vi "Controller.vi"() -> ()   [LabVIEW 2018]
uses:
  <vilib>/Platform/TimedLoop/XDataNode/timing_clust.ctl
  <vilib>/Platform/TimedLoop/XDataNode/nitl_modes.ctl
  <vilib>/Platform/TimedLoop/XDataNode/wakeup.ctl
  <vilib>/Modbus/master/Create Master Instance (TCP).vi
  <vilib>/Modbus/slave/Create Slave Instance (TCP).vi
  <vilib>/Modbus/master/Modbus Master.lvclass
  <vilib>/Platform/TimedLoop/XDataNode/XDataNode.xnode
  <vilib>/Platform/TimedLoop/XDataNode/XDNodeRunTimeDep.lvlib
  <vilib>/Modbus/slave/Modbus Slave.lvclass
panel:
  in  "stop":bool
  out "BPCS-10TY100":dbl format="%.2f"
  out "BPCS-10AY300":dbl
  out "BPCS-SIM-TX-ARRAY":dbl[](array[numeric])
  out "BPCS-10Y200":dbl format="%.2f"
  out "HMI-10HIC100":dbl
  out "HMI-10TIC100-SP":dbl
  out "HMI-10TIC100-KPID":dbl[](array[numeric])
  out "HMI-10HIC200":dbl
  out "HMI-10LIC200-SP":dbl
  out "HMI-10LIC200-KPID":dbl[](array[numeric])
  out "HMI-10HIC300":dbl
  out "HMI-10TIC100_MA":bool
  out "HMI-10LIC200_MA":bool
  out "SIS-BPCS-RX-Array":bool[](array[boolean])
  out "SIS-10SDV501":bool
  out "SIS-10SDV500":bool
  out "SIS-10SDV502":bool
  out "BPCS-10LI200":dbl
  out "SIM-BPCS-RX-ARRAY":dbl[](array[numeric])
  out "BPCS-10TI100":dbl
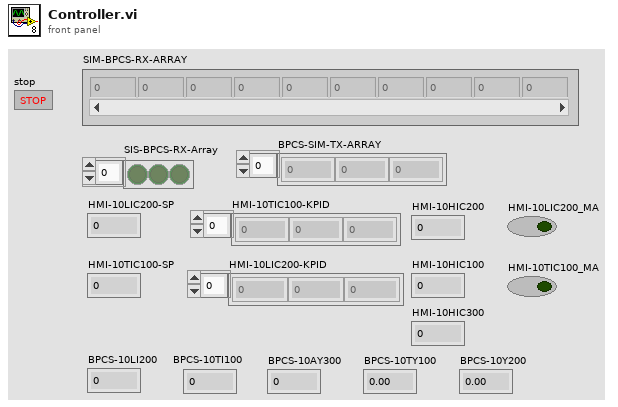
[diagram p1: front panel]
types:
  T1 = typedef "XDNodeRunTimeDep.lvlib/timing_clust.ctl" = cluster{"Expected End [f-1]":u64, "Actual End [f-1]":u64, "Finished Late? [f-1]":bool, "Expected End [i-1]":u64, "Actual End [i-1]":u64, "Finished Late? [i-1]":bool, "Expected Start [i]":u64, "Actual Start [i]":u64, "Expected Start [f]":u64, "Actual Start [f]":u64, "Source Name":string, "Structure Name":string, "Period":i64, "Deadline":i64, "Offset":i64, "Start":i64, "Priority":i32, "Timeout":i32, "Mode":T2, "Wakeup Reason":T3, "Error":errorcluster, "Source Type":string, "Secondary Source Type":string, "Global End Time":u64, "Global Start Time":u64, "Frame Duration":u64, "Iteration Duration":u64, "Assigned CPU":i32, "I/O Scan Engine Mode":u32}
  T2 = typedef "XDNodeRunTimeDep.lvlib/nitl_modes.ctl" = enum32{"No Change", "Process missed periods, maintain original phase", "Discard missed periods, maintain original phase", "Process missed periods, ignore original phase", "Discard missed periods, ignore original phase"}
  T3 = typedef "XDNodeRunTimeDep.lvlib/wakeup.ctl" = enum32{"Normal", "Aborted", "Asynchronous wakeup", "Timing source error", "Timed loop error", "Timeout"}
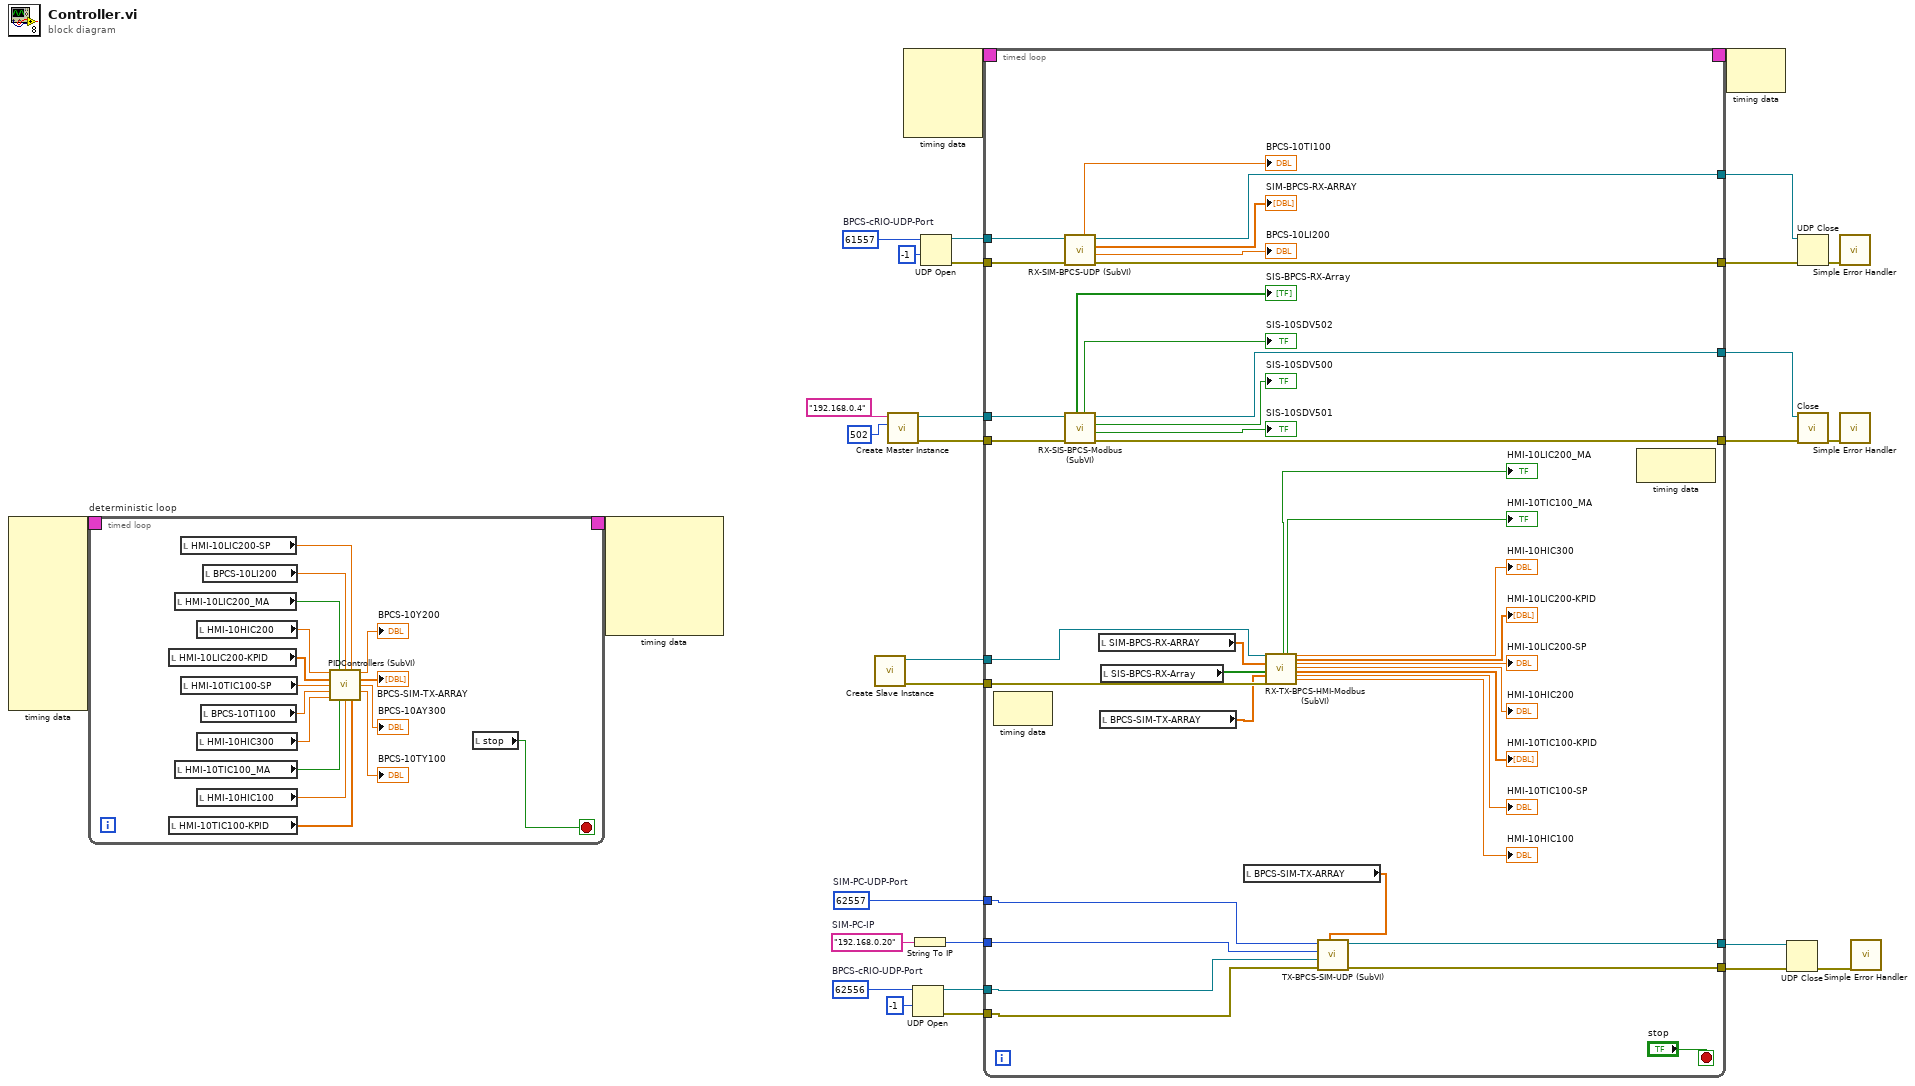
[diagram p0: block diagram]
diagram:
  w11 = u16 62556  # BPCS-cRIO-UDP-Port
  w9 = u16 62557  # SIM-PC-UDP-Port
  w12 = "192.168.0.20"  # SIM-PC-IP
  w28 = u16 61557  # BPCS-cRIO-UDP-Port
  n1 = node-c288 ("Input Node")() -> (w2:T1)  [unwired: 10 in]
  n2 = timed-loop "deterministic loop" {
    timing: w2 -> [_]
    timing-out: [_] -> w1
    stop <- w31 stop-if-true
    n3 = local read "HMI-10LIC200-KPID"() -> (w42:dbl[])
    n4 = local read "HMI-10TIC100-KPID"() -> (w36:dbl[])
    n5 = local read "HMI-10LIC200_MA"() -> (w44:bool)
    n6 = local read "HMI-10TIC100_MA"() -> (w38:bool)
    n7 = local read "HMI-10LIC200-SP"() -> (w46:dbl)
    n8 = local read "HMI-10TIC100-SP"() -> (w41:dbl)
    n9 = local read "HMI-10HIC200"() -> (w43:dbl)
    n10 = local read "HMI-10HIC300"() -> (w39:dbl)
    n11 = local read "HMI-10HIC100"() -> (w37:dbl)
    n12 = local read "BPCS-10TI100"() -> (w40:dbl)
    n13 = local read "BPCS-10LI200"() -> (w45:dbl)
    n14 = call "PIDControllers (SubVI).vi"("HMI-10HIC200"=w43, "HMI-10LIC200_MA"=w44, "BPCS-10LI200"=w45, "HMI-10LIC200-SP"=w46, "HMI-10LIC200-KPID"=w42, "HMI-10TIC100-SP"=w41, "BPCS-10TI100"=w40, "HMI-10HIC300"=w39, "HMI-10TIC100_MA"=w38, "HMI-10HIC100"=w37, "HMI-10TIC100-KPID"=w36) -> ("BPCS-10Y200"=→"BPCS-10Y200":dbl, "BPCS-SIM-TX-ARRAY"=→"BPCS-SIM-TX-ARRAY":dbl[], "BPCS-10AY300"=→"BPCS-10AY300":dbl, "BPCS-10TY100"=→"BPCS-10TY100":dbl)  [unwired: 1 in]
    n15 = local read "stop"() -> (w31:bool)
  }
  n16 = node-c288 ("Output Node")(w1) -> ()  [unwired: 6 out]
  n17 = call-poly <vilib>:"Create Slave Instance.vi"() -> ("error out"=w13:errorcluster, "TCP slave instance"=w14:refnum<class "Modbus Slave.lvclass">)  [unwired: 10 in]
  n18 = call-poly <vilib>:"Create Master Instance.vi"("port (502)"=u16 502, "address"="192.168.0.4") -> ("error out"=w18:errorcluster, "TCP master instance"=w19:refnum<class "Modbus Master.lvclass">)  [unwired: 8 in]
  n19 = node-c288() -> (w30:T1)  [unwired: 4 in]
  n20 = UDP Open(9:-1 ("timeout ms (25000)"), 11:w11) -> (port=w7:refnum<k16>, 0:w6:errorcluster)  [unwired: 3 in, 1 out]
  n21 = String To IP(1:w12) -> (0:w8:u32)
  n22 = UDP Open(9:-1 ("timeout ms (25000)"), 11:w28) -> (port=w26:refnum<k16>, 0:w25:errorcluster)  [unwired: 3 in, 1 out]
  n23 = timed-loop {
    timing: w30 -> [_]
    timing-out: [_] -> w29
    tunnel: w26 -> [w85]
    tunnel: w25 -> [w84]
    tunnel: [w83] -> w23
    tunnel: [w82] -> w22
    tunnel: w19 -> [w78]
    tunnel: w18 -> [w77]
    tunnel: [w76] -> w16
    tunnel: [w75] -> w15
    tunnel: w14 -> [w71]
    tunnel: w13 -> [w70]
    tunnel: w9 -> [w57]
    tunnel: w8 -> [w56]
    tunnel: w7 -> [w55]
    tunnel: w6 -> [w54]
    tunnel: [w53] -> w4
    tunnel: [w52] -> w3
    stop <- "stop" stop-if-true
    n24 = node-c288() -> ()  [unwired: 1 in, 1 out]
    n25 = call "RX-SIM-BPCS-UDP (SubVI).vi"("error in (no error)"=w84, "UDP Network Connection in"=w85) -> ("error out"=w82:errorcluster, "BPCS-10LI200"=→"BPCS-10LI200":dbl, "SIM-BPCS-RX-ARRAY"=→"SIM-BPCS-RX-ARRAY":dbl[], "UDP Network Connection out"=w83:refnum<k16>, "BPCS-10TI100"=→"BPCS-10TI100":dbl)  [unwired: 5 in]
    n26 = call "RX-SIS-BPCS-Modbus (SubVI).vi"("error in (no error)"=w77, "Modbus Master in"=w78) -> ("error out"=w75:errorcluster, "SIS-10SDV501"=→"SIS-10SDV501":bool, "SIS-10SDV500"=→"SIS-10SDV500":bool, "Modbus Master out"=w76:refnum<class "Modbus Master.lvclass">, "SIS-10SDV502"=→"SIS-10SDV502":bool, "SIS-BPCS-RX-Array"=→"SIS-BPCS-RX-Array":bool[])  [unwired: 4 in]
    n27 = local read "SIM-BPCS-RX-ARRAY"() -> (w68:dbl[])
    n28 = local read "BPCS-SIM-TX-ARRAY"() -> (w51:dbl[])
    n29 = local read "SIS-BPCS-RX-Array"() -> (w67:bool[])
    n30 = local read "BPCS-SIM-TX-ARRAY"() -> (w50:dbl[])
    n31 = call "RX-TX-BPCS-HMI-Modbus (SubVI).vi"("Modbus Slave in"=w71, "SIM-BPCS-RX-ARRAY"=w68, "SIS-BPCS-RX-Array"=w67, "BPCS-SIM-TX-ARRAY"=w51, "error in (no error)"=w70) -> ("HMI-10LIC200_MA"=→"HMI-10LIC200_MA":bool, "HMI-10TIC100_MA"=→"HMI-10TIC100_MA":bool, "HMI-10HIC300"=→"HMI-10HIC300":dbl, "HMI-10LIC200-KPID"=→"HMI-10LIC200-KPID":dbl[], "HMI-10LIC200-SP"=→"HMI-10LIC200-SP":dbl, "HMI-10HIC200"=→"HMI-10HIC200":dbl, "HMI-10TIC100-KPID"=→"HMI-10TIC100-KPID":dbl[], "HMI-10TIC100-SP"=→"HMI-10TIC100-SP":dbl, "HMI-10HIC100"=→"HMI-10HIC100":dbl)  [unwired: 14 in]
    n32 = call "TX-BPCS-SIM-UDP (SubVI).vi"("BPCS-SIM-TX-ARRAY in"=w50, "error in (no error)"=w54, "UDP Network Connection in"=w55, "SIM-PC-IP"=w56, "SIM-PC-UDP-Port"=w57) -> ("error out"=w52:errorcluster, "UDP Network Connection out"=w53:refnum<k16>)  [unwired: 3 in, 2 out]
    n33 = node-c288() -> ()  [unwired: 1 in, 1 out]
  }
  n34 = node-c288(w29) -> ()  [unwired: 1 out]
  n35 = UDP Close(connection ID=w4, 8:w3) -> (error out=w5:errorcluster)  [unwired: 1 out]
  n36 = UDP Close(connection ID=w23, 8:w22) -> (error out=w24:errorcluster)  [unwired: 1 out]
  n37 = call-dynamic "Close.vi"("error in (no error)"=w15, "Modbus master in"=w16) -> ("error out"=w17:errorcluster)  [unwired: 9 in]
  n38 = call <vilib>:"Simple Error Handler.vi"("error in (no error)"=w24) -> ()  [unwired: 4 in, 5 out]
  n39 = call <vilib>:"Simple Error Handler.vi"("error in (no error)"=w17) -> ()  [unwired: 4 in, 5 out]
  n40 = call <vilib>:"Simple Error Handler.vi"("error in (no error)"=w5) -> ()  [unwired: 4 in, 5 out]
